vi "PCO_GetCameraDescription3.vi"(8 "error in (no error)":errorcluster {"code" format="%x"}, 11 "ph":u64) -> (0 "error out":errorcluster {"code" format="%x"}, 1 "strDescription":T1, 2 "ErrorMessage":i32 format="%x", 3 "ph out":u64)   [LabVIEW 2019, in "SDK.lvlib" / "CameraDescription.lvlib"]
doc: "<b>Description:</b>\nAny of the available sensor and camera specific description can be queried. With input parameter wType the returned description structure can be selected. PCO_DescriptionEx is a generic structure which has to be casted to/from the queried structure. The wSize parameter has to be filled with the correct value for the requested structure. This function was introduced due to the size limitation of the standard camera descriptor and the need for describing additional features.\n\n<b>Supported camera type:</b>\nAll cameras\n\n<b>Descriptor dependency:</b>\ndwGeneralCapsDESC1: ENHANCED_DESCRIPTOR_2"
uses:
  CameraDescription.lvlib
  Structures/Structures.lvlib
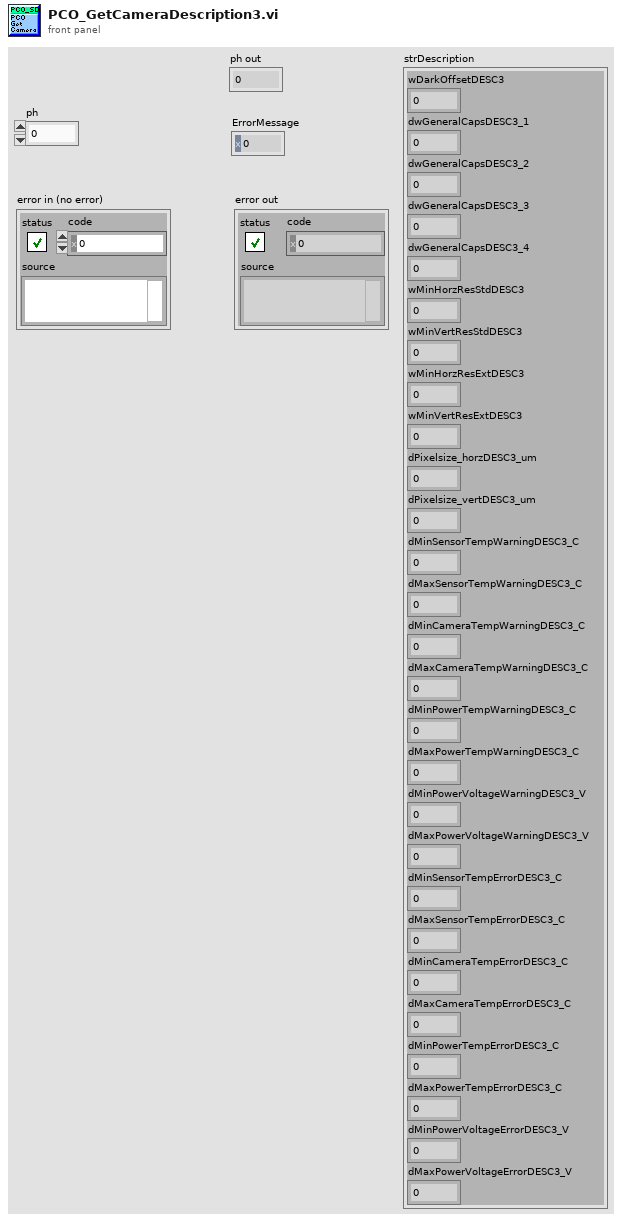
[diagram p1: front panel]
types:
  T1 = cluster{"wDarkOffsetDESC3":u16, "dwGeneralCapsDESC3_1":u32, "dwGeneralCapsDESC3_2":u32, "dwGeneralCapsDESC3_3":u32, "dwGeneralCapsDESC3_4":u32, "wMinHorzResStdDESC3":u16, "wMinVertResStdDESC3":u16, "wMinHorzResExtDESC3":u16, "wMinVertResExtDESC3":u16, "dPixelsize_horzDESC3_um":dbl, "dPixelsize_vertDESC3_um":dbl, "dMinSensorTempWarningDESC3_C":dbl, "dMaxSensorTempWarningDESC3_C":dbl, "dMinCameraTempWarningDESC3_C":dbl, "dMaxCameraTempWarningDESC3_C":dbl, "dMinPowerTempWarningDESC3_C":dbl, "dMaxPowerTempWarningDESC3_C":dbl, "dMinPowerVoltageWarningDESC3_V":dbl, "dMaxPowerVoltageWarningDESC3_V":dbl, "dMinSensorTempErrorDESC3_C":dbl, "dMaxSensorTempErrorDESC3_C":dbl, "dMinCameraTempErrorDESC3_C":dbl, "dMaxCameraTempErrorDESC3_C":dbl, "dMinPowerTempErrorDESC3_C":dbl, "dMaxPowerTempErrorDESC3_C":dbl, "dMinPowerVoltageErrorDESC3_V":dbl, "dMaxPowerVoltageErrorDESC3_V":dbl}
  T2 = cluster{"wSize":u16, "wDarkOffsetDESC3":u16, "dwGeneralCapsDESC3_1":u32, "dwGeneralCapsDESC3_2":u32, "dwGeneralCapsDESC3_3":u32, "dwGeneralCapsDESC3_4":u32, "wMinHorzResStdDESC3":u16, "wMinVertResStdDESC3":u16, "wMinHorzResExtDESC3":u16, "wMinVertResExtDESC3":u16, "wPixelsize_horzDESC3":u16, "wPixelsize_horzDESC3":u16, "sMinSensorTempWarningDESC3":i16, "sMaxSensorTempWarningDESC3":i16, "sMinCameraTempWarningDESC3":i16, "sMaxCameraTempWarningDESC3":i16, "sMinPowerTempWarningDESC3":i16, "sMaxPowerTempWarningDESC3":i16, "wMinPowerVoltageWarningDESC3":u16, "wMaxPowerVoltageWarningDESC3":u16, "sMinSensorTempErrorDESC3":i16, "sMaxSensorTempErrorDESC3":i16, "sMinCameraTempErrorDESC3":i16, "sMaxCameraTempErrorDESC3":i16, "sMinPowerTempErrorDESC3":i16, "sMaxPowerTempErrorDESC3":i16, "wMinPowerVoltageErrorDESC3":u16, "wMaxPowerVoltageErrorDESC3":u16, "dwReserved":cluster{u32, u32, u32, u32, u32, u32, u32, u32, u32, u32, u32, u32, u32, u32, u32, u32, u32, u32, u32, u32, u32, u32, u32, u32, u32, u32, u32, u32, u32, u32, u32, u32}}
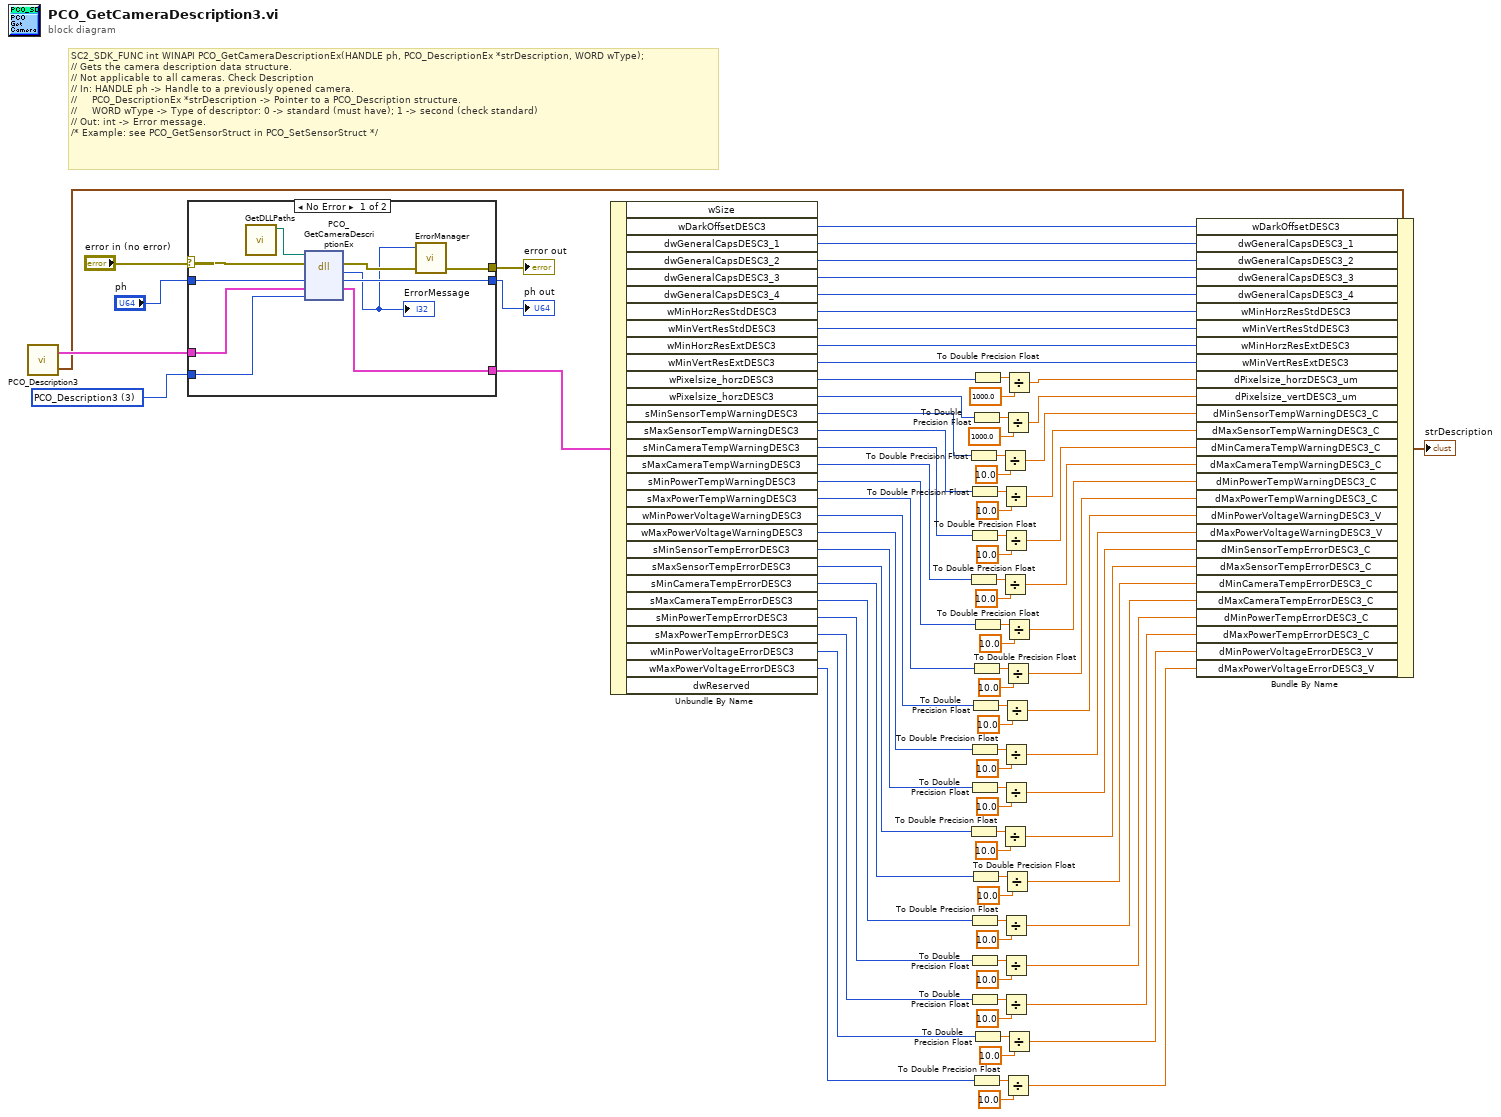
[diagram p0: block diagram]
diagram:
  w84 = u16 3 items=["PCO_Description", "PCO_Description2", "PCO_Description_Intensified", "PCO_Description3"] ("wType")
  # "SC2_SDK_FUNC int WINAPI PCO_GetCameraDescriptionEx(HANDLE ph, PCO_DescriptionEx *strDescription, WORD wType);\n// Gets the camera description data structure.\n// Not applicable to all cameras. Check Description\n// In: HANDLE ph -> Handle to a previously opened camera.\n//     PCO_DescriptionEx *strDescription -> Pointer to a PCO_Description structure.\n//     WORD wType -> Type of descriptor: 0 -> standard (must have); 1 -> second (check standard)\n// Out: int -> Error message.\n/* Example: see PCO_GetSensorStruct in PCO_SetSensorStruct */"
  n1 = call "PCO_Description3.vi"() -> ("PCO_Description3"=w83:T1, "PCO_Description3_Raw"=w86:T2)  [unwired: 4 in, 2 out]
  n2 = case shown="No Error" "error in (no error)" {
    selector: "error in (no error)" -> [w99 w103]
    tunnel: "ph" -> [w100 w102]
    tunnel: w86 -> [w94 w101]
    tunnel: [w96 w103] -> w88
    tunnel: [w98 w102] -> w87
    tunnel: [w93 w101] -> w85
    tunnel: w84 -> [w92 _]
    frame No Error {
      n3 = call "GetDLLPaths.vi"() -> ("SC2_Cam_Path"=w91:path)  [unwired: 9 in, 2 out]
      n4 = dll-call lib="?" fn="PCO_GetCameraDescriptionEx"(path in=w91, error in=w99, "ph"=w100, "strDescription"=w94, "wType"=w92) -> (error out=w97:errorcluster, "return type"=w95:i32, "ph"=w98:u64, "strDescription"=w93:T2)  [unwired: 2 in, 1 out]
      "ErrorMessage" <- w95
      n5 = call "ErrorManager.vi"("error in (no error)"=w97, "error code"=w95) -> ("error out"=w96:errorcluster)  [unwired: 3 in]
    }
    frame Error {
    }
  }
  "error out" <- w88
  "ph out" <- w87
  n6 = Unbundle By Name(w85) -> ("wDarkOffsetDESC3"=w81:u16, "dwGeneralCapsDESC3_1"=w80:u32, "dwGeneralCapsDESC3_2"=w79:u32, "dwGeneralCapsDESC3_3"=w78:u32, "dwGeneralCapsDESC3_4"=w77:u32, "wMinHorzResStdDESC3"=w76:u16, "wMinVertResStdDESC3"=w75:u16, "wMinHorzResExtDESC3"=w74:u16, "wMinVertResExtDESC3"=w73:u16, "wPixelsize_horzDESC3"=w36:u16, "wPixelsize_horzDESC3"=w35:u16, "sMinSensorTempWarningDESC3"=w34:i16, "sMaxSensorTempWarningDESC3"=w33:i16, "sMinCameraTempWarningDESC3"=w32:i16, "sMaxCameraTempWarningDESC3"=w31:i16, "sMinPowerTempWarningDESC3"=w30:i16, "sMaxPowerTempWarningDESC3"=w29:i16, "wMinPowerVoltageWarningDESC3"=w28:u16, "wMaxPowerVoltageWarningDESC3"=w27:u16, "sMinSensorTempErrorDESC3"=w26:i16, "sMaxSensorTempErrorDESC3"=w25:i16, "sMinCameraTempErrorDESC3"=w24:i16, "sMaxCameraTempErrorDESC3"=w23:i16, "sMinPowerTempErrorDESC3"=w22:i16, "sMaxPowerTempErrorDESC3"=w21:i16, "wMinPowerVoltageErrorDESC3"=w20:u16, "wMaxPowerVoltageErrorDESC3"=w19:u16)  [unwired: 2 out]
  n7 = To Double Precision Float(number=w34) -> (double precision float=w67:dbl)
  n8 = To Double Precision Float(number=w31) -> (double precision float=w61:dbl)
  n9 = To Double Precision Float(number=w25) -> (double precision float=w49:dbl)
  n10 = To Double Precision Float(number=w33) -> (double precision float=w65:dbl)
  n11 = To Double Precision Float(number=w32) -> (double precision float=w63:dbl)
  n12 = To Double Precision Float(number=w27) -> (double precision float=w53:dbl)
  n13 = To Double Precision Float(number=w26) -> (double precision float=w51:dbl)
  n14 = To Double Precision Float(number=w23) -> (double precision float=w45:dbl)
  n15 = To Double Precision Float(number=w22) -> (double precision float=w43:dbl)
  n16 = To Double Precision Float(number=w21) -> (double precision float=w41:dbl)
  n17 = To Double Precision Float(number=w28) -> (double precision float=w55:dbl)
  n18 = To Double Precision Float(number=w24) -> (double precision float=w47:dbl)
  n19 = To Double Precision Float(number=w35) -> (double precision float=w69:dbl)
  n20 = To Double Precision Float(number=w29) -> (double precision float=w57:dbl)
  n21 = To Double Precision Float(number=w19) -> (double precision float=w37:dbl)
  n22 = To Double Precision Float(number=w36) -> (double precision float=w72:dbl)
  n23 = To Double Precision Float(number=w30) -> (double precision float=w59:dbl)
  n24 = To Double Precision Float(number=w20) -> (double precision float=w39:dbl)
  n25 = Divide(x=w67, y=10.0) -> (x/y=w16:dbl)
  n26 = Divide(x=w61, y=10.0) -> (x/y=w13:dbl)
  n27 = Divide(x=w49, y=10.0) -> (x/y=w7:dbl)
  n28 = Divide(x=w65, y=10.0) -> (x/y=w15:dbl)
  n29 = Divide(x=w63, y=10.0) -> (x/y=w14:dbl)
  n30 = Divide(x=w53, y=10.0) -> (x/y=w9:dbl)
  n31 = Divide(x=w51, y=10.0) -> (x/y=w8:dbl)
  n32 = Divide(x=w45, y=10.0) -> (x/y=w5:dbl)
  n33 = Divide(x=w43, y=10.0) -> (x/y=w4:dbl)
  n34 = Divide(x=w41, y=10.0) -> (x/y=w3:dbl)
  n35 = Divide(x=w55, y=10.0) -> (x/y=w10:dbl)
  n36 = Divide(x=w47, y=10.0) -> (x/y=w6:dbl)
  n37 = Divide(x=w69, y=1000.0) -> (x/y=w17:dbl)
  n38 = Divide(x=w57, y=10.0) -> (x/y=w11:dbl)
  n39 = Divide(x=w37, y=10.0) -> (x/y=w1:dbl)
  n40 = Divide(x=w72, y=1000.0) -> (x/y=w18:dbl)
  n41 = Divide(x=w59, y=10.0) -> (x/y=w12:dbl)
  n42 = Divide(x=w39, y=10.0) -> (x/y=w2:dbl)
  n43 = Bundle By Name(cluster=w83, "wDarkOffsetDESC3"=w81, "dwGeneralCapsDESC3_1"=w80, "dwGeneralCapsDESC3_2"=w79, "dwGeneralCapsDESC3_3"=w78, "dwGeneralCapsDESC3_4"=w77, "wMinHorzResStdDESC3"=w76, "wMinVertResStdDESC3"=w75, "wMinHorzResExtDESC3"=w74, "wMinVertResExtDESC3"=w73, "dPixelsize_horzDESC3_um"=w18, "dPixelsize_vertDESC3_um"=w17, "dMinSensorTempWarningDESC3_C"=w16, "dMaxSensorTempWarningDESC3_C"=w15, "dMinCameraTempWarningDESC3_C"=w14, "dMaxCameraTempWarningDESC3_C"=w13, "dMinPowerTempWarningDESC3_C"=w12, "dMaxPowerTempWarningDESC3_C"=w11, "dMinPowerVoltageWarningDESC3_V"=w10, "dMaxPowerVoltageWarningDESC3_V"=w9, "dMinSensorTempErrorDESC3_C"=w8, "dMaxSensorTempErrorDESC3_C"=w7, "dMinCameraTempErrorDESC3_C"=w6, "dMaxCameraTempErrorDESC3_C"=w5, "dMinPowerTempErrorDESC3_C"=w4, "dMaxPowerTempErrorDESC3_C"=w3, "dMinPowerVoltageErrorDESC3_V"=w2, "dMaxPowerVoltageErrorDESC3_V"=w1) -> (→"strDescription":T1)
